vi "Initialize Buffer.vi"(4 "Error In":errorcluster, 7 "Instance Name":T1) -> (0 "Error Out":errorcluster)   [LabVIEW 2015, in "Temperature Controller Data Buffer.lvlib"]
uses:
  Temperature Controller Data Buffer.lvlib
  _libraries/Startup Processes/_typedefs/Subpanel Names.ctl
  _libraries/Config Data/Config Data.lvclass
  _libraries/Startup Processes/Startup Processes.lvlib
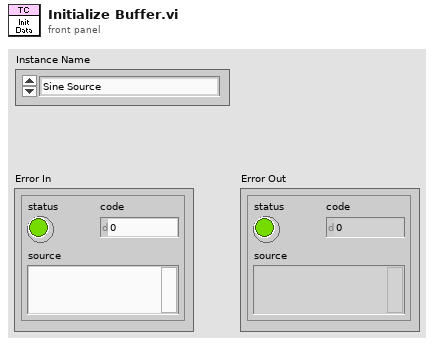
[diagram p1: front panel]
types:
  T1 = typedef "Startup Processes.lvlib/Subpanel Names.ctl" = enum16{"Sine Source", "Ramp Source", "Hen House TC", "Dog House TC", "Out House TC"}
  T2 = typedef "Temperature Controller Data Buffer.lvlib/buffer data typedef.ctl" = cluster{"TC Data":cluster{"Last value":dbl, "Error High Level":dbl, "Warning High Level":dbl, "Warning Low Level":dbl, "Error Low Level":dbl}[], "Counter":i32}
  T3 = cluster{"Last value":dbl, "Error High Level":dbl, "Warning High Level":dbl, "Warning Low Level":dbl, "Error Low Level":dbl}[]
  T4 = cluster{"Last value":dbl, "Error High Level":dbl, "Warning High Level":dbl, "Warning Low Level":dbl, "Error Low Level":dbl}
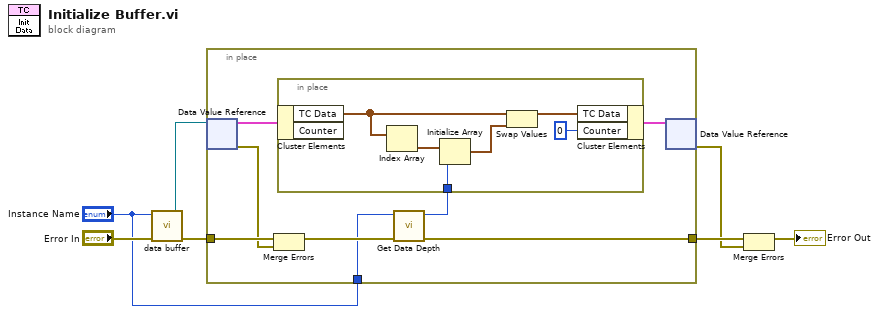
[diagram p0: block diagram]
diagram:
  n1 = call "data buffer.vi"("Error In"="Error In", "Instance Name"="Instance Name") -> ("Error Out"=w5:errorcluster, "DVR"=w6:refnum<data-value>)  [unwired: 4 in]
  n2 = in-place {
    in-place-border: w5 -> [w15]
    in-place-border: [w12] -> w4
    in-place-border: "Instance Name" -> [w8]
    n3 = in-place-dvr #1(w6) -> (w11:T2, w14:errorcluster)
    n4 = Merge Errors(w15, w14) -> (w13:errorcluster)
    n5 = call "Get Data Depth.vi"("error in (no error)"=w13, "Depth to fetch"=w8) -> ("error out"=w12:errorcluster, "Data Depth"=w10:i32)  [unwired: 4 in]
    n6 = in-place {
      in-place-border: w10 -> [w21]
      n7 = in-place-cluster #2(w11) -> ("TC Data"=w18:T3)  [unwired: 1 out]
      n8 = Index Array(array=w18) -> (element=w19:T4)  [unwired: 1 in]
      n9 = Initialize Array(w19, w21) -> (w20:T3)
      n10 = Swap Values(12:w18, 14:w20) -> (1:w17:T3)  [unwired: 1 in, 1 out]
      n11 = in-place-cluster #2("TC Data"=w17, "Counter"=0) -> (w9:T2)
    }
    n12 = in-place-dvr #1(w9) -> (w2:errorcluster)  [unwired: 1 out]
  }
  n13 = Merge Errors(w4, w2) -> (→"Error Out":errorcluster)
